vi "AlGaInPAs_prep_run_cont_v05.vi"(2 "Debug Mode":bool, 3 "Elapsed Time(s)":dbl, 4 "State":enum16{"Edit", "Start", "Run", "End", "Idle"}(ring), 5 "Argument List In":string[](array[string])) -> (0 "Status Out":string, 1 "Argument List Out":string[](array[string]))   [LabVIEW 2011]
panel:
  out "total time":dbl
  out "is OK?":bool
  out "AsH3?":bool
  out "PH3?":bool
  out "In?":bool
  out "Ga?":bool
  out "Al?":bool
  in  "Prep As":bool caption="Pre-run"
  in  "Prep P":bool caption="Pre-run"
  in  "Prep In":bool caption="Pre-run"
  in  "Prep Ga":bool caption="Pre-run"
  in  "prep_time":dbl caption="pre-run time (s)"
  in  "Prep Al":bool caption="Pre-run"
  in  "Run As":bool caption="Run"
  in  "AsH3 Flow":dbl caption="AsH3 Flow (0-10 sccm)" format="%.2f"
  in  "P Flow":dbl caption="P Flow (0-100 sccm)" format="%.2f"
  in  "Run P":bool caption="Run"
  in  "In Flow":dbl caption="In Flow (0-100 sscm)" format="%.2f"
  in  "Run In":bool caption="Run"
  in  "Run Ga":bool caption="Run"
  in  "Ga Flow":dbl caption="Ga Flow (0-10 sscm)" format="%.2f"
  in  "Run Al":bool caption="Run"
  in  "Al Flow":dbl caption="Al Flow (0-100 sscm)" format="%.2f"
  in  "Cancel":bool
  in  "OK":bool
  out "tTotal(s) 2":dbl
  # "Add pre-run time to run time in editor."
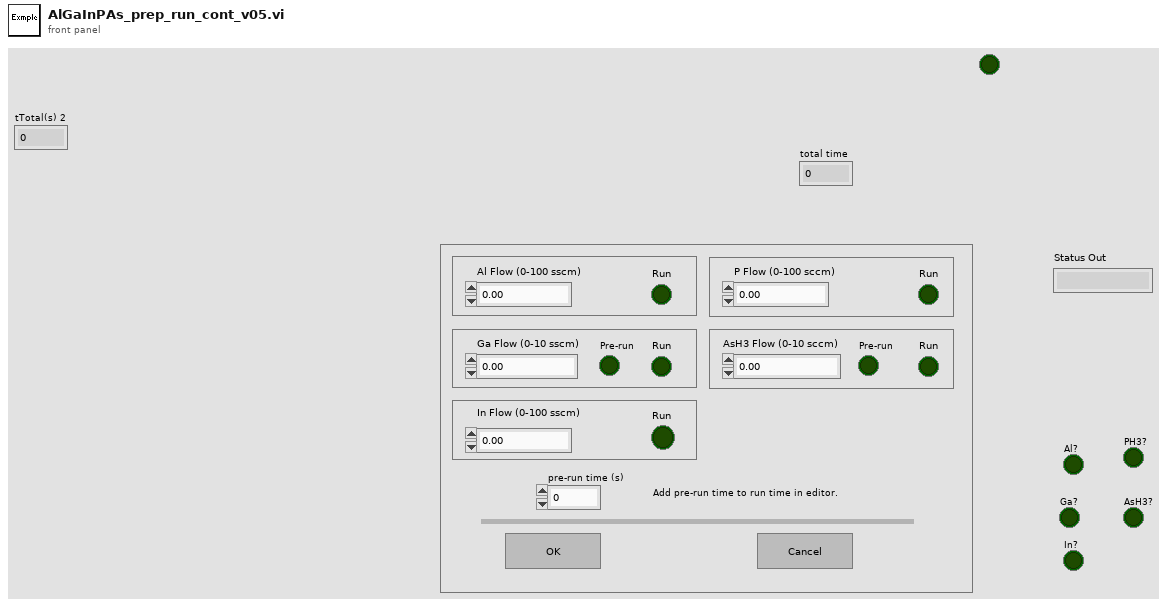
[diagram p1: front panel]
types:
  T1 = enum16{"Discrete", "Continuous", "Instantaneous"}
  T2 = enum32{"Invalid", "Default", "Floating", "Floating/Auto-Hide", "Modal"}
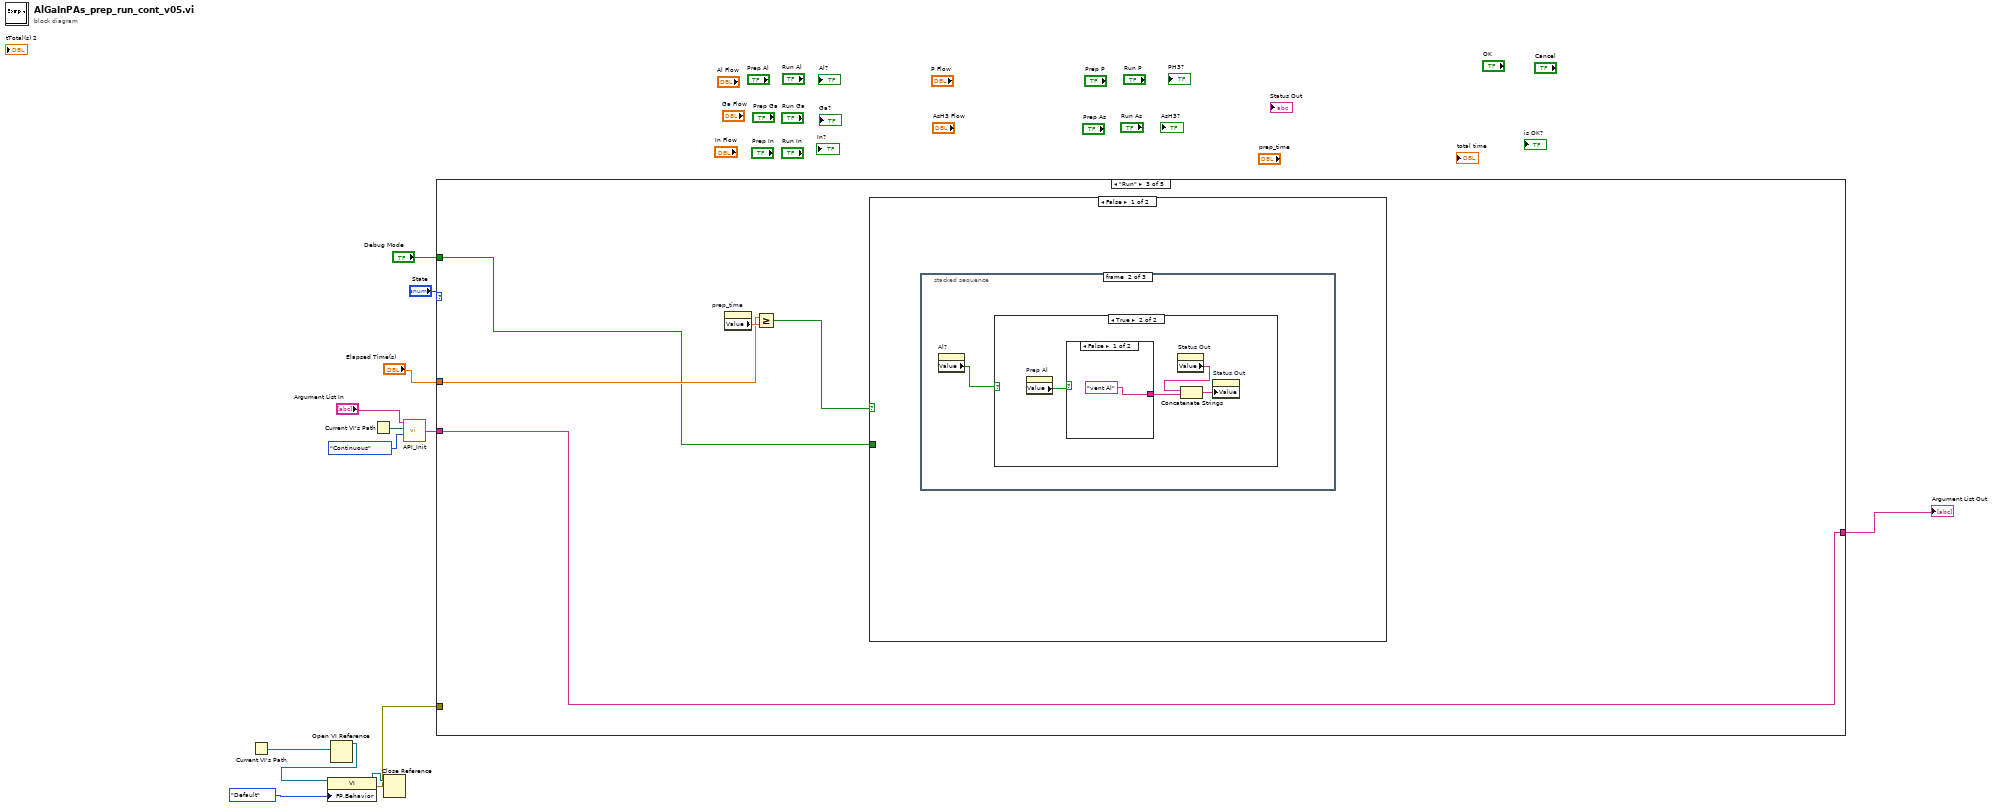
[diagram p0: block diagram]
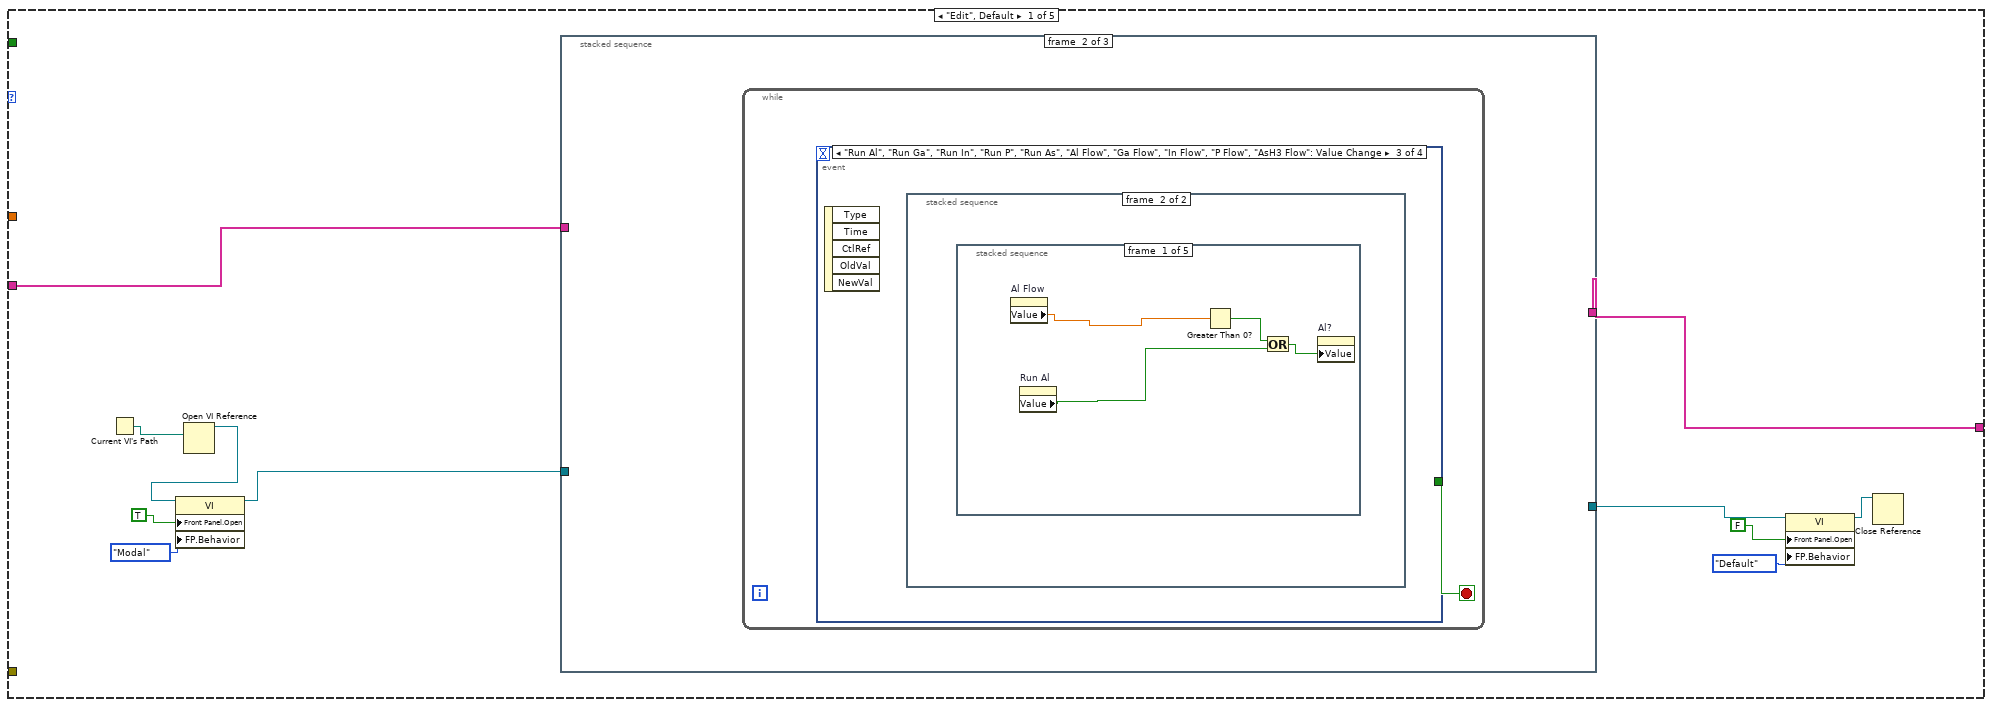
[diagram p2: hidden frame]
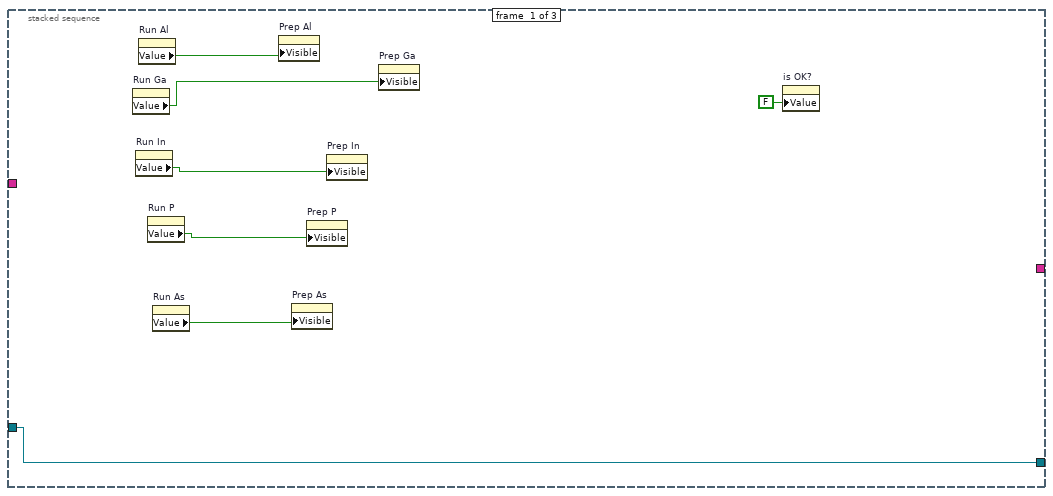
[diagram p3: hidden frame]
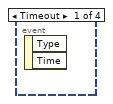
[diagram p4: hidden frame]
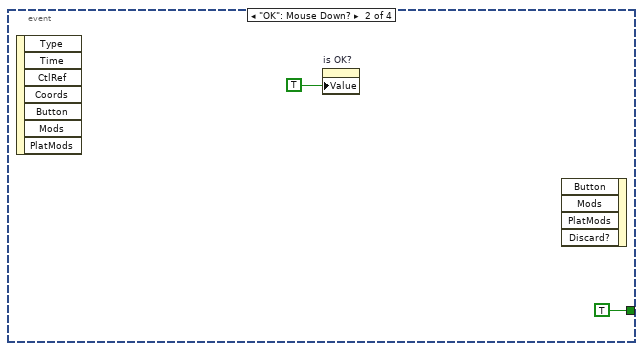
[diagram p5: hidden frame]
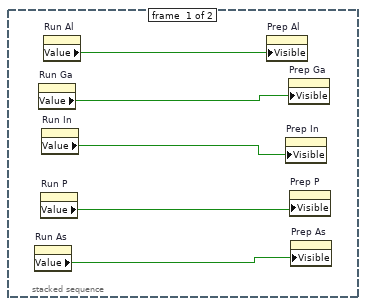
[diagram p6: hidden frame]
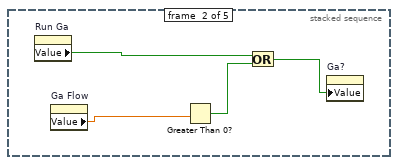
[diagram p7: hidden frame]
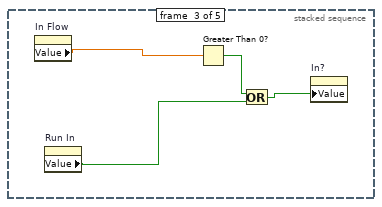
[diagram p8: hidden frame]
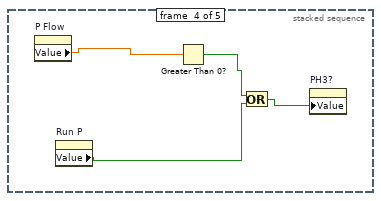
[diagram p9: hidden frame]
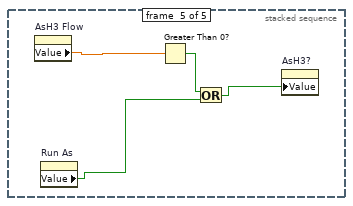
[diagram p10: hidden frame]
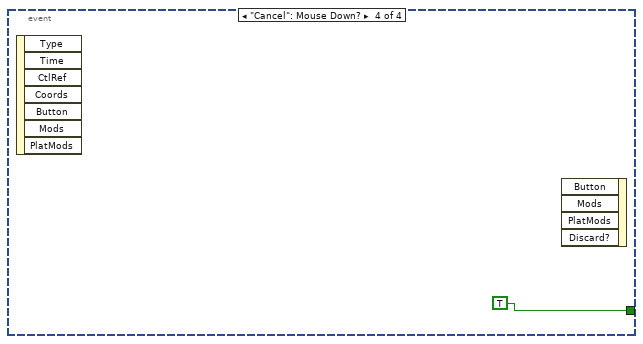
[diagram p11: hidden frame]
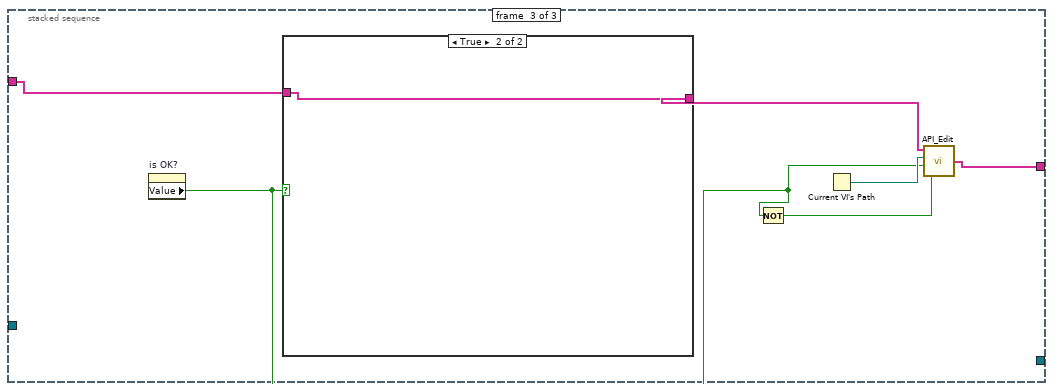
[diagram p12: hidden frame]
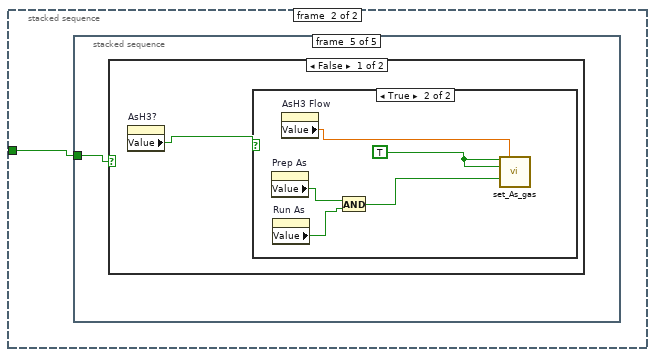
[diagram p15: hidden frame]
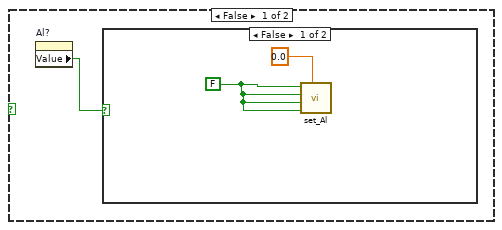
[diagram p17: hidden frame]
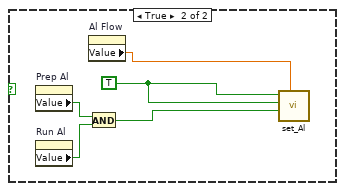
[diagram p18: hidden frame]
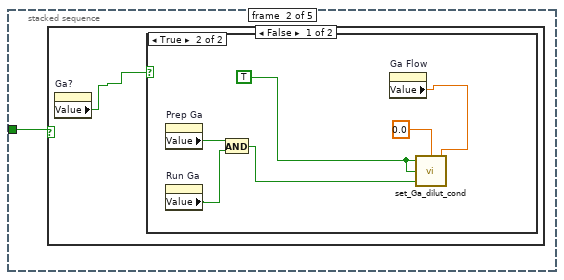
[diagram p19: hidden frame]
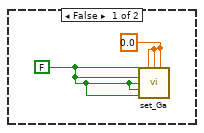
[diagram p20: hidden frame]
diagram:
  n1 = Current VI's Path() -> (path=w9:path)
  n2 = Open VI Reference(vi path=w9) -> (vi reference=w8:refnum<vi>)  [unwired: 1 in, 5 out]
  n3 = property class="VI"(reference=w8, "FP.Behavior"=T2."Default" ("Front Panel Window:Behavior")) -> (reference out=w6:refnum<vi>, error out=w5:errorcluster)  [unwired: 1 in]
  n4 = Current VI's Path() -> (path=w4:path)
  n5 = Close Reference(reference=w6) -> ()  [unwired: 1 in, 1 out]
  n6 = call "API_Init.vi"("API Mode"=T1."Continuous", "VI Path"=w4, "Argument List In"="Argument List In") -> ("Argument List Out"=w1:string[])  [unwired: 1 in]
  n7 = case shown="\"Run\"" "State" {
    tunnel: "Debug Mode" -> [_ w69 w119 _ _]
    tunnel: "Elapsed Time(s)" -> [_ _ w120 _ _]
    tunnel: w1 -> [w15 w70 w122 w182 w183]
    tunnel: [w14 w70 w122 w182 w183] -> w10
    tunnel: w5 -> [_ _ _ _ _]
    frame "Edit", Default {
      n8 = Current VI's Path() -> (path=w20:path)
      n9 = Open VI Reference(vi path=w20) -> (vi reference=w19:refnum<vi>)  [unwired: 1 in, 5 out]
      n10 = property class="VI"(reference=w19, "Front Panel.Open"=TRUE ("Front Panel Window:Open"), "FP.Behavior"=T2."Modal" ("Front Panel Window:Behavior")) -> (reference out=w18:refnum<vi>)  [unwired: 1 in, 1 out]
      n11 = stacked-sequence {
        tunnel: w15 -> [_ _ w64]
        tunnel: w18 -> [w31 _ _]
        tunnel: [w31 _ _] -> w22
        tunnel: [_ _ w62] -> w14
        frame #0 {
          n12 = property on="Run Ga" class="Bool (strict)"() -> ("Value"=w28:bool)  [unwired: 2 in, 2 out]
          n13 = property on="Run In" class="Bool (strict)"() -> ("Value"=w27:bool)  [unwired: 2 in, 2 out]
          n14 = property on="Run Al" class="Bool (strict)"() -> ("Value"=w29:bool)  [unwired: 2 in, 2 out]
          n15 = property on="Run P" class="Bool (strict)"() -> ("Value"=w26:bool)  [unwired: 2 in, 2 out]
          n16 = property on="Run As" class="Bool (strict)"() -> ("Value"=w25:bool)  [unwired: 2 in, 2 out]
          n17 = property on="Prep Al" class="Bool (strict)"("Visible"=w29) -> ()  [unwired: 2 in, 2 out]
          n18 = property on="Prep As" class="Bool (strict)"("Visible"=w25) -> ()  [unwired: 2 in, 2 out]
          n19 = property on="Prep P" class="Bool (strict)"("Visible"=w26) -> ()  [unwired: 2 in, 2 out]
          n20 = property on="Prep In" class="Bool (strict)"("Visible"=w27) -> ()  [unwired: 2 in, 2 out]
          n21 = property on="Prep Ga" class="Bool (strict)"("Visible"=w28) -> ()  [unwired: 2 in, 2 out]
          n22 = property on="is OK?" class="Bool (strict)"("Value"=FALSE ("is OK?")) -> ()  [unwired: 2 in, 2 out]
        }
        frame #1 {
          n23 = while {
            stop <- w32 stop-if-true
            n24 = event shown="[2] \"Run Al\", \"Run Ga\", \"Run In\", \"Run P\", \"Run As\", \"Al Flow\", \"Ga Flow\", \"In Flow\", \"P Flow\", \"AsH3 Flow\": Value Change" {
              selector: _ -> [_ _ _ _]
              dyn-events: _ -> [_ _ _ _]
              timeout: _ -> [_ _ _ _]
              tunnel: [_ TRUE _ TRUE] -> w32
              event Timeout {
                n25 = event-data() -> ()  [unwired: 1 in, 2 out]
              }
              event "OK": Mouse Down? {
                n26 = event-data() -> ()  [unwired: 1 in, 7 out]
                n27 = property on="is OK?" class="Bool (strict)"("Value"=TRUE ("is OK?")) -> ()  [unwired: 2 in, 2 out]
                n28 = event-data() -> ()  [unwired: 5 in, 1 out]
              }
              event "Run Al", "Run Ga", "Run In", "Run P", "Run As", "Al Flow", "Ga Flow", "In Flow", "P Flow", "AsH3 Flow": Value Change {
                n29 = event-data() -> ()  [unwired: 1 in, 5 out]
                n30 = stacked-sequence {
                  frame #0 {
                    n31 = property on="Run As" class="Bool (strict)"() -> ("Value"=w35:bool)  [unwired: 2 in, 2 out]
                    n32 = property on="Run Ga" class="Bool (strict)"() -> ("Value"=w38:bool)  [unwired: 2 in, 2 out]
                    n33 = property on="Run P" class="Bool (strict)"() -> ("Value"=w36:bool)  [unwired: 2 in, 2 out]
                    n34 = property on="Run In" class="Bool (strict)"() -> ("Value"=w37:bool)  [unwired: 2 in, 2 out]
                    n35 = property on="Run Al" class="Bool (strict)"() -> ("Value"=w39:bool)  [unwired: 2 in, 2 out]
                    n36 = property on="Prep Al" class="Bool (strict)"("Visible"=w39) -> ()  [unwired: 2 in, 2 out]
                    n37 = property on="Prep In" class="Bool (strict)"("Visible"=w37) -> ()  [unwired: 2 in, 2 out]
                    n38 = property on="Prep Ga" class="Bool (strict)"("Visible"=w38) -> ()  [unwired: 2 in, 2 out]
                    n39 = property on="Prep P" class="Bool (strict)"("Visible"=w36) -> ()  [unwired: 2 in, 2 out]
                    n40 = property on="Prep As" class="Bool (strict)"("Visible"=w35) -> ()  [unwired: 2 in, 2 out]
                  }
                  frame #1 {
                    n41 = stacked-sequence {
                      frame #0 {
                        n42 = property on="Al Flow" class="DigNum (strict)"() -> ("Value"=w42:dbl)  [unwired: 2 in, 2 out]
                        n43 = property on="Run Al" class="Bool (strict)"() -> ("Value"=w41:bool)  [unwired: 2 in, 2 out]
                        n44 = Greater Than 0?(x=w42) -> (x > 0?=w43:bool)
                        n45 = Or(x=w43, y=w41) -> (x .or. y?=w40:bool)
                        n46 = property on="Al?" class="Bool (strict)"("Value"=w40) -> ()  [unwired: 2 in, 2 out]
                      }
                      frame #1 {
                        n47 = property on="Run Ga" class="Bool (strict)"() -> ("Value"=w45:bool)  [unwired: 2 in, 2 out]
                        n48 = property on="Ga Flow" class="DigNum (strict)"() -> ("Value"=w46:dbl)  [unwired: 2 in, 2 out]
                        n49 = Greater Than 0?(x=w46) -> (x > 0?=w47:bool)
                        n50 = Or(x=w45, y=w47) -> (x .or. y?=w44:bool)
                        n51 = property on="Ga?" class="Bool (strict)"("Value"=w44) -> ()  [unwired: 2 in, 2 out]
                      }
                      frame #2 {
                        n52 = property on="In Flow" class="DigNum (strict)"() -> ("Value"=w49:dbl)  [unwired: 2 in, 2 out]
                        n53 = property on="Run In" class="Bool (strict)"() -> ("Value"=w50:bool)  [unwired: 2 in, 2 out]
                        n54 = Greater Than 0?(x=w49) -> (x > 0?=w51:bool)
                        n55 = Or(x=w51, y=w50) -> (x .or. y?=w48:bool)
                        n56 = property on="In?" class="Bool (strict)"("Value"=w48) -> ()  [unwired: 2 in, 2 out]
                      }
                      frame #3 {
                        n57 = property on="P Flow" class="DigNum (strict)"() -> ("Value"=w54:dbl)  [unwired: 2 in, 2 out]
                        n58 = property on="Run P" class="Bool (strict)"() -> ("Value"=w53:bool)  [unwired: 2 in, 2 out]
                        n59 = Greater Than 0?(x=w54) -> (x > 0?=w55:bool)
                        n60 = Or(x=w55, y=w53) -> (x .or. y?=w52:bool)
                        n61 = property on="PH3?" class="Bool (strict)"("Value"=w52) -> ()  [unwired: 2 in, 2 out]
                      }
                      frame #4 {
                        n62 = property on="AsH3 Flow" class="DigNum (strict)"() -> ("Value"=w58:dbl)  [unwired: 2 in, 2 out]
                        n63 = property on="Run As" class="Bool (strict)"() -> ("Value"=w57:bool)  [unwired: 2 in, 2 out]
                        n64 = Greater Than 0?(x=w58) -> (x > 0?=w59:bool)
                        n65 = Or(x=w59, y=w57) -> (x .or. y?=w56:bool)
                        n66 = property on="AsH3?" class="Bool (strict)"("Value"=w56) -> ()  [unwired: 2 in, 2 out]
                      }
                    }
                  }
                }
              }
              event "Cancel": Mouse Down? {
                n67 = event-data() -> ()  [unwired: 1 in, 7 out]
                n68 = event-data() -> ()  [unwired: 5 in, 1 out]
              }
            }
          }
        }
        frame #2 {
          n69 = property on="is OK?" class="Bool (strict)"() -> ("Value"=w61:bool)  [unwired: 2 in, 2 out]
          n70 = case shown="True" w61 {
            tunnel: w64 -> [w67 w68]
            tunnel: [w67 w68] -> w63
            frame False {
            }
            frame True {
            }
          }
          n71 = Not(x=w61) -> (.not. x?=w66:bool)
          n72 = Current VI's Path() -> (path=w65:path)
          n73 = call "API_Edit.vi"("Cancel"=w66, "OK"=w61, "VI Path"=w65, "Argument List In"=w63) -> ("Argument List Out"=w62:string[])
        }
      }
      n74 = property class="VI"(reference=w22, "Front Panel.Open"=FALSE ("Front Panel Window:Open"), "FP.Behavior"=T2."Default" ("Front Panel Window:Behavior")) -> (reference out=w23:refnum<vi>)  [unwired: 1 in, 1 out]
      n75 = Close Reference(reference=w23) -> ()  [unwired: 1 in, 1 out]
    }
    frame "Start" {
      n76 = stacked-sequence {
        tunnel: w69 -> [_ w71]
        frame #0 {
        }
        frame #1 {
          n77 = stacked-sequence {
            tunnel: w71 -> [w72 w81 w91 w100 w109]
            frame #0 {
              n78 = case shown="True" w72 {
                frame False {
                  n79 = property on="Al?" class="Bool (strict)"() -> ("Value"=w73:bool)  [unwired: 2 in, 2 out]
                  n80 = case shown="False" w73 {
                    frame False {
                      w74 = FALSE ("Al Active")
                      n81 = call "set_Al.vi"("Aluminum Flow"=0.0, "Al Remote"=w74, "Al Run"=w74, "Al Bubbler"=w74, "Al Active"=w74) -> ()  [unwired: 5 out]
                    }
                    frame True {
                      w80 = TRUE ("Al Active")
                      n82 = property on="Prep Al" class="Bool (strict)"() -> ("Value"=w78:bool)  [unwired: 2 in, 2 out]
                      n83 = property on="Run Al" class="Bool (strict)"() -> ("Value"=w77:bool)  [unwired: 2 in, 2 out]
                      n84 = property on="Al Flow" class="DigNum (strict)"() -> ("Value"=w79:dbl)  [unwired: 2 in, 2 out]
                      n85 = And(x=w78, y=w77) -> (x .and. y?=w76:bool)
                      n86 = call "set_Al.vi"("Aluminum Flow"=w79, "Al Run"=w76, "Al Bubbler"=w80, "Al Active"=w80) -> ()  [unwired: 1 in, 5 out]
                    }
                  }
                }
                frame True {
                }
              }
            }
            frame #1 {
              n87 = case shown="False" w81 {
                frame False {
                  n88 = property on="Ga?" class="Bool (strict)"() -> ("Value"=w82:bool)  [unwired: 2 in, 2 out]
                  n89 = case shown="True" w82 {
                    frame False {
                      w84 = FALSE ("Ga Active")
                      w83 = 0.0 ("Ga Flow 1")
                      n90 = call "set_Ga.vi"("Ga Active"=w84, "Ga Flow 3"=w83, "Ga Flow 2"=w83, "Ga Flow 1"=w83, "Ga Bubbler"=w84, "Ga H2 Dilute"=w84, "Ga Run"=w84, "Ga Remote"=w84) -> ()  [unwired: 8 out]
                    }
                    frame True {
                      w90 = TRUE ("Ga Active")
                      n91 = property on="Prep Ga" class="Bool (strict)"() -> ("Value"=w87:bool)  [unwired: 2 in, 2 out]
                      n92 = property on="Run Ga" class="Bool (strict)"() -> ("Value"=w86:bool)  [unwired: 2 in, 2 out]
                      n93 = And(x=w87, y=w86) -> (x .and. y?=w85:bool)
                      n94 = property on="Ga Flow" class="DigNum (strict)"() -> ("Value"=w88:dbl)  [unwired: 2 in, 2 out]
                      n95 = call "set_Ga_dilut_cond.vi"("Ga flow (0-10 sccm)"=w88, "fDilution"=0.0, "Run"=w85, "Bubbler In"=w90, "Active"=w90) -> ()
                    }
                  }
                }
                frame True {
                }
              }
            }
            frame #2 {
              n96 = case shown="False" w91 {
                frame False {
                  n97 = property on="In?" class="Bool (strict)"() -> ("Value"=w92:bool)  [unwired: 2 in, 2 out]
                  n98 = case shown="True" w92 {
                    frame False {
                      w94 = FALSE ("In Remote")
                      n99 = call "set_In.vi"("Indium Flow"=0.0, "In Remote"=w94, "In Run"=w94, "In Bubbler"=w94, "In Active"=w94) -> ()  [unwired: 5 out]
                    }
                    frame True {
                      w99 = TRUE ("In Run")
                      n100 = property on="Run In" class="Bool (strict)"() -> ("Value"=w96:bool)  [unwired: 2 in, 2 out]
                      n101 = property on="Prep In" class="Bool (strict)"() -> ("Value"=w97:bool)  [unwired: 2 in, 2 out]
                      n102 = And(x=w97, y=w96) -> (x .and. y?=w95:bool)
                      n103 = property on="In Flow" class="DigNum (strict)"() -> ("Value"=w98:dbl)  [unwired: 2 in, 2 out]
                      n104 = call "set_In.vi"("Indium Flow"=w98, "In Run"=w95, "In Bubbler"=w99, "In Active"=w99) -> ()  [unwired: 1 in, 5 out]
                    }
                  }
                }
                frame True {
                }
              }
            }
            frame #3 {
              n105 = case shown="False" w100 {
                frame False {
                  n106 = property on="PH3?" class="Bool (strict)"() -> ("Value"=w101:bool)  [unwired: 2 in, 2 out]
                  n107 = case shown="True" w101 {
                    frame False {
                      w102 = FALSE ("P_Gas Active")
                      n108 = call "set_P_gas.vi"("P_Gas Active"=w102, "P_Gas Flow"=0.0, "P_Gas In"=w102, "P_Gas H2 In"=w102, "P_Gas Run"=w102, "P_Gas Remote"=w102) -> ()  [unwired: 10 out]
                    }
                    frame True {
                      w108 = TRUE ("P_Gas Active")
                      n109 = property on="P Flow" class="DigNum (strict)"() -> ("Value"=w107:dbl)  [unwired: 2 in, 2 out]
                      n110 = property on="Prep P" class="Bool (strict)"() -> ("Value"=w106:bool)  [unwired: 2 in, 2 out]
                      n111 = property on="Run P" class="Bool (strict)"() -> ("Value"=w105:bool)  [unwired: 2 in, 2 out]
                      n112 = And(x=w106, y=w105) -> (x .and. y?=w104:bool)
                      n113 = call "set_P_gas.vi"("P_Gas Active"=w108, "P_Gas Flow"=w107, "P_Gas In"=w108, "P_Gas Run"=w104) -> ()  [unwired: 2 in, 10 out]
                    }
                  }
                }
                frame True {
                }
              }
            }
            frame #4 {
              n114 = case shown="False" w109 {
                frame False {
                  n115 = property on="AsH3?" class="Bool (strict)"() -> ("Value"=w110:bool)  [unwired: 2 in, 2 out]
                  n116 = case shown="True" w110 {
                    frame False {
                      w111 = FALSE ("As_Gas Active")
                      n117 = call "set_As_gas.vi"("As_Gas Active"=w111, "As_Gas Flow"=0.0, "As_Gas In"=w111, "As_Gas H2"=w111, "As_Gas Run"=w111, "As_Gas Remote"=w111) -> ()  [unwired: 10 in]
                    }
                    frame True {
                      w117 = TRUE ("As_Gas Active")
                      n118 = property on="Prep As" class="Bool (strict)"() -> ("Value"=w114:bool)  [unwired: 2 in, 2 out]
                      n119 = property on="Run As" class="Bool (strict)"() -> ("Value"=w115:bool)  [unwired: 2 in, 2 out]
                      n120 = property on="AsH3 Flow" class="DigNum (strict)"() -> ("Value"=w116:dbl)  [unwired: 2 in, 2 out]
                      n121 = And(x=w114, y=w115) -> (x .and. y?=w113:bool)
                      n122 = call "set_As_gas.vi"("As_Gas Active"=w117, "As_Gas Flow"=w116, "As_Gas In"=w117, "As_Gas Run"=w113) -> ()  [unwired: 12 in]
                    }
                  }
                }
                frame True {
                }
              }
            }
          }
        }
      }
    }
    frame "Run" {
      n123 = property on="prep_time" class="DigNum (strict)"() -> ("Value"=w121:dbl)  [unwired: 2 in, 2 out]
      n124 = Greater Or Equal?(x=w120, y=w121) -> (x >= y?=w118:bool)
      n125 = case shown="False" w118 {
        tunnel: w119 -> [_ w143]
        frame False {
          n126 = stacked-sequence {
            frame #0 {
              n127 = property on="Status Out" class="Str"("Value"="prep:") -> ()  [unwired: 2 in, 2 out]
            }
            frame #1 {
              n128 = property on="Al?" class="Bool (strict)"() -> ("Value"=w124:bool)  [unwired: 2 in, 2 out]
              n129 = case shown="True" w124 {
                frame False {
                  w125 = ""
                }
                frame True {
                  n130 = property on="Prep Al" class="Bool (strict)"() -> ("Value"=w129:bool)  [unwired: 2 in, 2 out]
                  n131 = case shown="False" w129 {
                    tunnel: ["vent Al" "run Al"] -> w126
                    frame False {
                    }
                    frame True {
                    }
                  }
                  n132 = property on="Status Out" class="Str"() -> ("Value"=w127:string)  [unwired: 2 in, 2 out]
                  n133 = Concatenate Strings(w127, w126) -> (w128:string)
                  n134 = property on="Status Out" class="Str"("Value"=w128) -> ()  [unwired: 2 in, 2 out]
                }
              }
            }
            frame #2 {
              n135 = property on="AsH3?" class="Bool (strict)"() -> ("Value"=w132:bool)  [unwired: 2 in, 2 out]
              n136 = case shown="True" w132 {
                frame False {
                }
                frame True {
                  n137 = property on="Prep As" class="Bool (strict)"() -> ("Value"=w136:bool)  [unwired: 2 in, 2 out]
                  n138 = case shown="True" w136 {
                    tunnel: ["vent As" "run As"] -> w135
                    frame False {
                    }
                    frame True {
                    }
                  }
                  n139 = property on="Status Out" class="Str"() -> ("Value"=w134:string)  [unwired: 2 in, 2 out]
                  n140 = Concatenate Strings(w134, w135) -> (w133:string)
                  n141 = property on="Status Out" class="Str"("Value"=w133) -> ()  [unwired: 2 in, 2 out]
                }
              }
            }
          }
        }
        frame True {
          n142 = stacked-sequence {
            tunnel: w143 -> [w146 w153 w161 w168 w175]
            frame #0 {
              n143 = case shown="False" w146 {
                frame False {
                  n144 = property on="Al?" class="Bool (strict)"() -> ("Value"=w147:bool)  [unwired: 2 in, 2 out]
                  n145 = case shown="True" w147 {
                    frame False {
                      w148 = FALSE ("Al Active")
                      n146 = call "set_Al.vi"("Aluminum Flow"=0.0, "Al Remote"=w148, "Al Run"=w148, "Al Bubbler"=w148, "Al Active"=w148) -> ()  [unwired: 5 out]
                    }
                    frame True {
                      w152 = TRUE ("Al Active")
                      n147 = property on="Al Flow" class="DigNum (strict)"() -> ("Value"=w151:dbl)  [unwired: 2 in, 2 out]
                      n148 = property on="Run Al" class="Bool (strict)"() -> ("Value"=w150:bool)  [unwired: 2 in, 2 out]
                      n149 = call "set_Al.vi"("Aluminum Flow"=w151, "Al Run"=w150, "Al Bubbler"=w152, "Al Active"=w152) -> ()  [unwired: 1 in, 5 out]
                    }
                  }
                }
                frame True {
                }
              }
            }
            frame #1 {
              n150 = case shown="False" w153 {
                frame False {
                  n151 = property on="Ga?" class="Bool (strict)"() -> ("Value"=w154:bool)  [unwired: 2 in, 2 out]
                  n152 = case shown="False" w154 {
                    frame False {
                      w156 = FALSE ("Ga Active")
                      w155 = 0.0 ("Ga Flow 1")
                      n153 = call "set_Ga.vi"("Ga Active"=w156, "Ga Flow 3"=w155, "Ga Flow 2"=w155, "Ga Flow 1"=w155, "Ga Bubbler"=w156, "Ga H2 Dilute"=w156, "Ga Run"=w156, "Ga Remote"=w156) -> ()  [unwired: 8 out]
                    }
                    frame True {
                      w160 = TRUE ("Ga Active")
                      n154 = property on="Ga Flow" class="DigNum (strict)"() -> ("Value"=w157:dbl)  [unwired: 2 in, 2 out]
                      n155 = property on="Run Ga" class="Bool (strict)"() -> ("Value"=w158:bool)  [unwired: 2 in, 2 out]
                      n156 = call "set_Ga_dilut_cond.vi"("Ga flow (0-10 sccm)"=w157, "fDilution"=0.0, "Run"=w158, "Bubbler In"=w160, "Active"=w160) -> ()
                    }
                  }
                }
                frame True {
                }
              }
            }
            frame #2 {
              n157 = case shown="False" w161 {
                frame False {
                  n158 = property on="In?" class="Bool (strict)"() -> ("Value"=w162:bool)  [unwired: 2 in, 2 out]
                  n159 = case shown="True" w162 {
                    frame False {
                      w164 = FALSE ("In Remote")
                      n160 = call "set_In.vi"("Indium Flow"=0.0, "In Remote"=w164, "In Run"=w164, "In Bubbler"=w164, "In Active"=w164) -> ()  [unwired: 5 out]
                    }
                    frame True {
                      w167 = TRUE ("In Run")
                      n161 = property on="Run In" class="Bool (strict)"() -> ("Value"=w165:bool)  [unwired: 2 in, 2 out]
                      n162 = property on="In Flow" class="DigNum (strict)"() -> ("Value"=w166:dbl)  [unwired: 2 in, 2 out]
                      n163 = call "set_In.vi"("Indium Flow"=w166, "In Run"=w165, "In Bubbler"=w167, "In Active"=w167) -> ()  [unwired: 1 in, 5 out]
                    }
                  }
                }
                frame True {
                }
              }
            }
            frame #3 {
              n164 = case shown="False" w168 {
                frame False {
                  n165 = property on="PH3?" class="Bool (strict)"() -> ("Value"=w169:bool)  [unwired: 2 in, 2 out]
                  n166 = case shown="False" w169 {
                    frame False {
                      w170 = FALSE ("P_Gas Active")
                      n167 = call "set_P_gas.vi"("P_Gas Active"=w170, "P_Gas Flow"=0.0, "P_Gas In"=w170, "P_Gas H2 In"=w170, "P_Gas Run"=w170, "P_Gas Remote"=w170) -> ()  [unwired: 10 out]
                    }
                    frame True {
                      w174 = TRUE ("P_Gas Active")
                      n168 = property on="P Flow" class="DigNum (strict)"() -> ("Value"=w173:dbl)  [unwired: 2 in, 2 out]
                      n169 = property on="Run P" class="Bool (strict)"() -> ("Value"=w172:bool)  [unwired: 2 in, 2 out]
                      n170 = call "set_P_gas.vi"("P_Gas Active"=w174, "P_Gas Flow"=w173, "P_Gas In"=w174, "P_Gas Run"=w172) -> ()  [unwired: 2 in, 10 out]
                    }
                  }
                }
                frame True {
                }
              }
            }
            frame #4 {
              n171 = case shown="False" w175 {
                frame False {
                  n172 = property on="AsH3?" class="Bool (strict)"() -> ("Value"=w176:bool)  [unwired: 2 in, 2 out]
                  n173 = case shown="False" w176 {
                    frame False {
                      w177 = FALSE ("As_Gas Active")
                      n174 = call "set_As_gas.vi"("As_Gas Active"=w177, "As_Gas Flow"=0.0, "As_Gas In"=w177, "As_Gas H2"=w177, "As_Gas Run"=w177, "As_Gas Remote"=w177) -> ()  [unwired: 10 in]
                    }
                    frame True {
                      w180 = TRUE ("As_Gas Active")
                      n175 = property on="Run As" class="Bool (strict)"() -> ("Value"=w179:bool)  [unwired: 2 in, 2 out]
                      n176 = property on="AsH3 Flow" class="DigNum (strict)"() -> ("Value"=w181:dbl)  [unwired: 2 in, 2 out]
                      n177 = call "set_As_gas.vi"("As_Gas Active"=w180, "As_Gas Flow"=w181, "As_Gas In"=w180, "As_Gas Run"=w179) -> ()  [unwired: 12 in]
                    }
                  }
                }
                frame True {
                }
              }
            }
          }
          n178 = property on="AsH3?" class="Bool (strict)"() -> ("Value"=w139:bool)  [unwired: 2 in, 2 out]
          n179 = case shown="False" w139 {
            tunnel: ["no As" "As"] -> w140
            frame False {
            }
            frame True {
            }
          }
          n180 = Concatenate Strings("run started" ("Status Out"), w140) -> (w142:string)
          n181 = property on="Status Out" class="Str"("Value"=w142) -> ()  [unwired: 2 in, 2 out]
        }
      }
    }
    frame "End" {
    }
    frame "Idle" {
    }
  }
  "Argument List Out" <- w10
